vi "32[2]-Trace Data Collection.vi"(8 "error in (no error)":errorcluster, 11 "32[2]-Trace Data Collection Data":T2) -> (0 "error out":errorcluster, 2 "Timeout?":bool, 3 "S2F24":T1)   [LabVIEW 2020, in "SECS Scenarios.lvlib" / "Scenarios Class.lvclass"]
uses:
  Scenarios Class.lvclass
  SECS Communication/S2 Message Class/S2F24.ctl
  32[2]-Trace Data Collection.ctl
  SECS Communication/S2 Message Class/S2 Message Class.lvclass
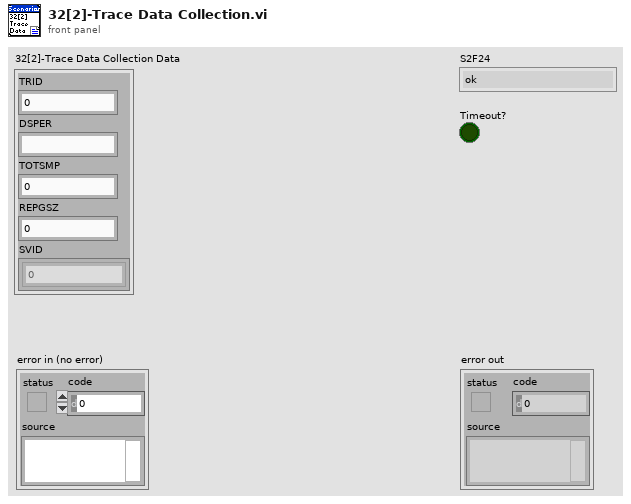
[diagram p1: front panel]
types:
  T1 = typedef "SECS Communication.lvlib/S2 Message Class.lvclass/S2F24.ctl" = enum16{"ok", "too many SVIDs", "no more traces allowed", "invalid period", "unknown SVID", "bad REPGSZ"}
  T2 = cluster{"TRID":u32, "DSPER":string, "TOTSMP":u32, "REPGSZ":u32, "SVID":u32[]}
  T3 = typedef "SECS Scenarios.lvlib/Scenarios Class.lvclass/32[2]-Trace Data Collection.ctl" = cluster{"TRID":u32, "DSPER":string, "TOTSMP":u32, "REPGSZ":u32, "SVID":u32[], "Reply Notifier":refnum<notifier>}
  T4 = typedef "SECS Scenarios.lvlib/Scenarios Class.lvclass/Broadcast Refnum.ctl" = cluster{"13-EnableDisable Alarm":refnum<user-event>, "15-Process Program Request":refnum<user-event>, "16-Process Program Send":refnum<user-event>, "17-Deleting a Process Program by Host":refnum<user-event>, "18-Host Requests Equipment Process Program Directory":refnum<user-event>, "19-Equipment Process Program Uploading":refnum<user-event>, "20[1]-Process Program Downloading":refnum<user-event>, "20[2]-Process Program Downloading":refnum<user-event>, "22-Host Sends Information to Equipment":refnum<user-event>, "26-Host Requests to Enter OFF-Line":refnum<user-event>, "27-Host Requests to Enter On-Line":refnum<user-event>, "28[1]-Remote Control[PP-SELECT]":refnum<user-event>, "28[2]-Remote Control[START]":refnum<user-event>, "28[3]-Remote Control[STOP]":refnum<user-event>, "28[4]-Remote Control[LOCAL]":refnum<user-event>, "28[5]-Remote Control[REMOTE]":refnum<user-event>, "28[6]-Remote Control[RCMD]":refnum<user-event>, "30-Host Requests Equipment to Set Time":refnum<user-event>, "31-Host Requests Time Value from Equipment":refnum<user-event>, "32[1]-Trace Data Collection":refnum<user-event>, "32[2]-Trace Data Collection":refnum<user-event>}
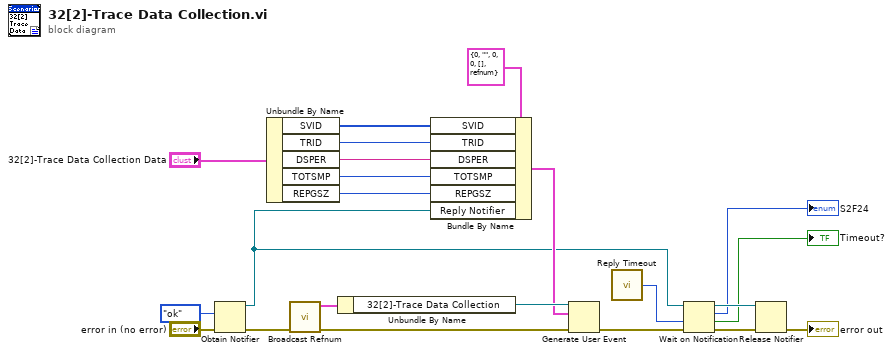
[diagram p0: block diagram]
diagram:
  n1 = Obtain Notifier(notification data type=S2F24."ok" ("S2F24"), error in (no error)="error in (no error)") -> (notifier out=w5:refnum<notifier>, error out=w10:errorcluster)  [unwired: 2 in, 1 out]
  n2 = Unbundle By Name("32[2]-Trace Data Collection Data") -> ("SVID"=w1:u32[], "TRID"=w16:u32, "DSPER"=w15:string, "TOTSMP"=w14:u32, "REPGSZ"=w13:u32)
  n3 = call "Broadcast Refnum.vi"("error in"=w10) -> ("error out"=w21:errorcluster, "Broadcast Refnum"=w22:T4)  [unwired: 9 in]
  n4 = Unbundle By Name(w22) -> ("32[2]-Trace Data Collection"=w20:refnum<user-event>)
  n5 = Bundle By Name(cluster=T3 {"TRID"=0, "DSPER"="", "TOTSMP"=0, "REPGSZ"=0, "SVID"=[], "Reply Notifier"=refnum} ("32[2]-Trace Data Collection"), "SVID"=w1, "TRID"=w16, "DSPER"=w15, "TOTSMP"=w14, "REPGSZ"=w13, "Reply Notifier"=w5) -> (w19:T3)
  n6 = Generate User Event(user event=w20, event data cluster=w19, error in=w21) -> (error out=w6:errorcluster)  [unwired: 1 in, 1 out]
  n7 = call "Reply Timeout.vi"() -> ("Reply Timeout"=w9:i32)
  n8 = Wait on Notification(notifier=w5, timeout in ms (-1)=w9, error in (no error)=w6) -> (notifier out=w8:refnum<notifier>, notification=→"S2F24":T1, timed out?=→"Timeout?":bool, error out=w7:errorcluster)  [unwired: 1 in]
  n9 = Release Notifier(notifier=w8, error in (no error)=w7) -> (error out=→"error out":errorcluster)  [unwired: 1 in, 2 out]
